vi "Dequeue Message.vi"(8 "error in (no error)":errorcluster, 11 "Message Queue":refnum<queue>) -> (0 "error out":errorcluster, 1 "Argument":string, 2 "Message":string, 3 "dup Message Queue":refnum<queue>, 4 "Message Data":variant, 6 "element":T1)   [LabVIEW 2013, in "Message Queue.lvlib"]
doc: "This VI pulls messages off the Message Queue."
uses:
  Message Queue.lvlib
  Message Cluster.ctl
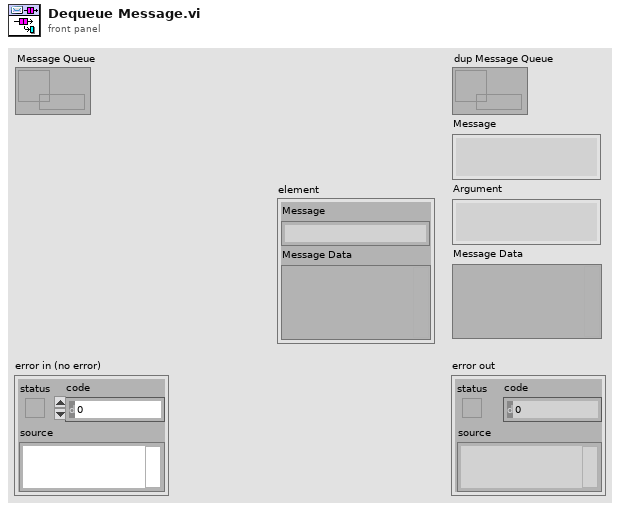
[diagram p1: front panel]
types:
  T1 = typedef "Message Queue.lvlib/Message Cluster.ctl" = cluster{"Message":string, "Message Data":variant}
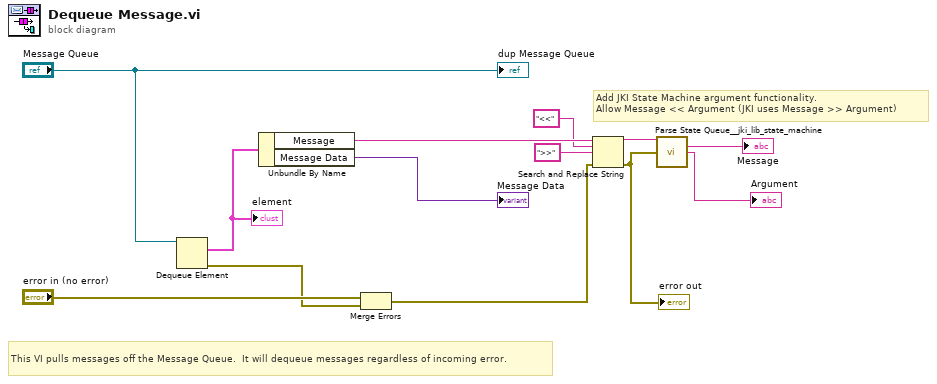
[diagram p0: block diagram]
diagram:
  # "Add JKI State Machine argument functionality.\nAllow Message << Argument (JKI uses Message >> Argument)"
  # "This VI pulls messages off the Message Queue.  It will dequeue messages regardless of incoming error."
  n1 = Dequeue Element(queue="Message Queue") -> (element=w11:T1, error out=w9:errorcluster)  [unwired: 2 in, 2 out]
  "element" <- w11
  n2 = Unbundle By Name(w11) -> ("Message"=w8:string, "Message Data"=→"Message Data":variant)
  n3 = Merge Errors("error in (no error)", w9) -> (w2:errorcluster)
  n4 = Search and Replace String(input string=w8, search string="<<", replace string=">>" ("replace string (\"\")"), error in=w2) -> (result string=w5:string, error out=w1:errorcluster)  [unwired: 4 in, 2 out]
  "error out" <- w1
  n5 = call <vilib>:"Parse State Queue__jki_lib_state_machine.vi"("State Queue"=w5, "Error In (no error)"=w1) -> ("Current State"=→"Message":string, "Arguments"=→"Argument":string)  [unwired: 11 in, 1 out]
  "dup Message Queue" <- "Message Queue"
